vi "Area.vi"(8 "error in (no error)":errorcluster, 11 "Picture2D in":refnum<class "Picture2D.lvclass">) -> (0 "error out":errorcluster, 2 "Area":T1, 3 "Picture2D out":refnum<class "Picture2D.lvclass">)   [LabVIEW 2021, in "Picture2D.lvlib" / "Picture2D.lvclass"]
uses:
  Picture2D.lvclass
  Picture2D.lvclass/Picture2D.ctl
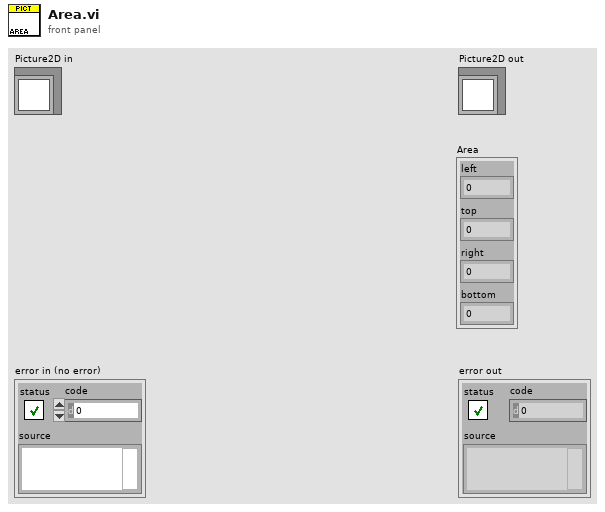
[diagram p1: front panel]
types:
  T1 = cluster{"left":i16, "top":i16, "right":i16, "bottom":i16}
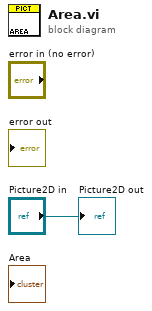
[diagram p0: block diagram]
diagram:
  "Picture2D out" <- "Picture2D in"
